vi "Send Default ILC Outputs.vi"(8 "error in (no error)":errorcluster, 11 "Model in":refnum<class "Model.lvclass">) -> (0 "error out":errorcluster, 3 "Model out":refnum<class "Model.lvclass">)   [LabVIEW 2015, in "Model.lvclass"]
uses:
  Model.lvclass
  <userlib>/Common/ILC/ILC/ILC.lvclass
  Actuator/Actuator/Actuator.lvclass
  Typedefs/Actuate Arguments.ctl
  Typedefs/FAMT Typedefs.lvlib
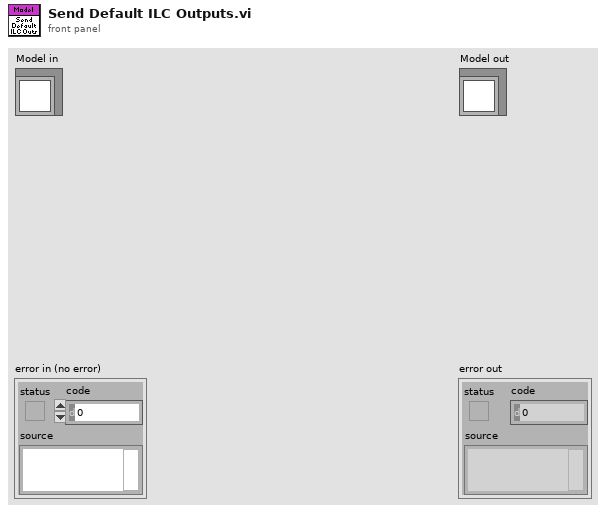
[diagram p1: front panel]
types:
  T1 = typedef "FAMT Typedefs.lvlib/Actuate Arguments.ctl" = cluster{"Axial Demand":dbl, "Lateral Demand":dbl, "FC1 Measured Value":dbl[unit], "FC2 Measured Value":dbl[unit]}
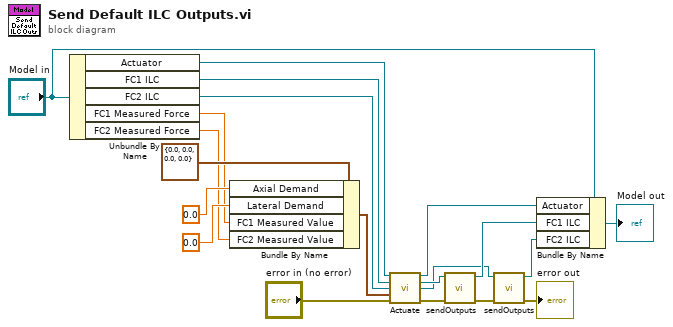
[diagram p0: block diagram]
diagram:
  n1 = Unbundle By Name("Model in") -> ("Actuator"=w2:refnum<class "Actuator.lvclass">, "FC1 ILC"=w10:refnum<class "ILC.lvclass">, "FC2 ILC"=w9:refnum<class "ILC.lvclass">, "FC1 Measured Force"=w4:dbl[unit], "FC2 Measured Force"=w3:dbl[unit])
  n2 = Bundle By Name(cluster=T1 {"Axial Demand"=0.0, "Lateral Demand"=0.0, "FC1 Measured Value"=0.0, "FC2 Measured Value"=0.0} ("Actuate Arguments"), "Axial Demand"=0.0, "Lateral Demand"=0.0, "FC1 Measured Value"=w4, "FC2 Measured Value"=w3) -> (w7:T1)
  n3 = call-dynamic "Actuate.vi"("Actuator in"=w2, "FC1 ILC in"=w10, "FC2 ILC in"=w9, "Actuate Arguments"=w7, "error in (no error)"="error in (no error)") -> ("Actuator out"=w1:refnum<class "Actuator.lvclass">, "FC1 ILC out"=w18:refnum<class "ILC.lvclass">, "FC2 ILC out"=w14:refnum<class "ILC.lvclass">, "error out"=w16:errorcluster)  [unwired: 7 in]
  n4 = call <userlib>:"sendOutputs.vi"("error in (no error)"=w16, "ILC in"=w18) -> ("error out"=w12:errorcluster, "ILC out"=w15:refnum<class "ILC.lvclass">)  [unwired: 8 in]
  n5 = call <userlib>:"sendOutputs.vi"("error in (no error)"=w12, "ILC in"=w14) -> ("error out"=→"error out":errorcluster, "ILC out"=w13:refnum<class "ILC.lvclass">)  [unwired: 8 in]
  n6 = Bundle By Name(cluster="Model in", "Actuator"=w1, "FC1 ILC"=w15, "FC2 ILC"=w13) -> (→"Model out":refnum<class "Model.lvclass">)
